vi "GUI_Frog_HPD_imagetested2.vi"() -> ()   [LabVIEW 2013]
uses:
  Shared/GUI_Template/GUI_master/tcp_new_data_event.ctl
  Shared/GUI_Template/GUI_master/tcp new data cluster.ctl
panel:
  out "tcp data event":T1
  in  "Refresh Button":bool
  in  "Select device":string(combo)="PL1-PresCtl"
  in  "triggermode::1":bool caption="Blank Button"
  out "retrievedFrogTrace::1":T2(plugin-control) caption="Retrieved Frog Trace"
  out "frogTrace::1":T2(plugin-control) caption="FROG Trace"
  in  "insert tag":bool=TRUE
  in  "stop":bool
  in  "GUIdevice 1":string="FrogHPD"
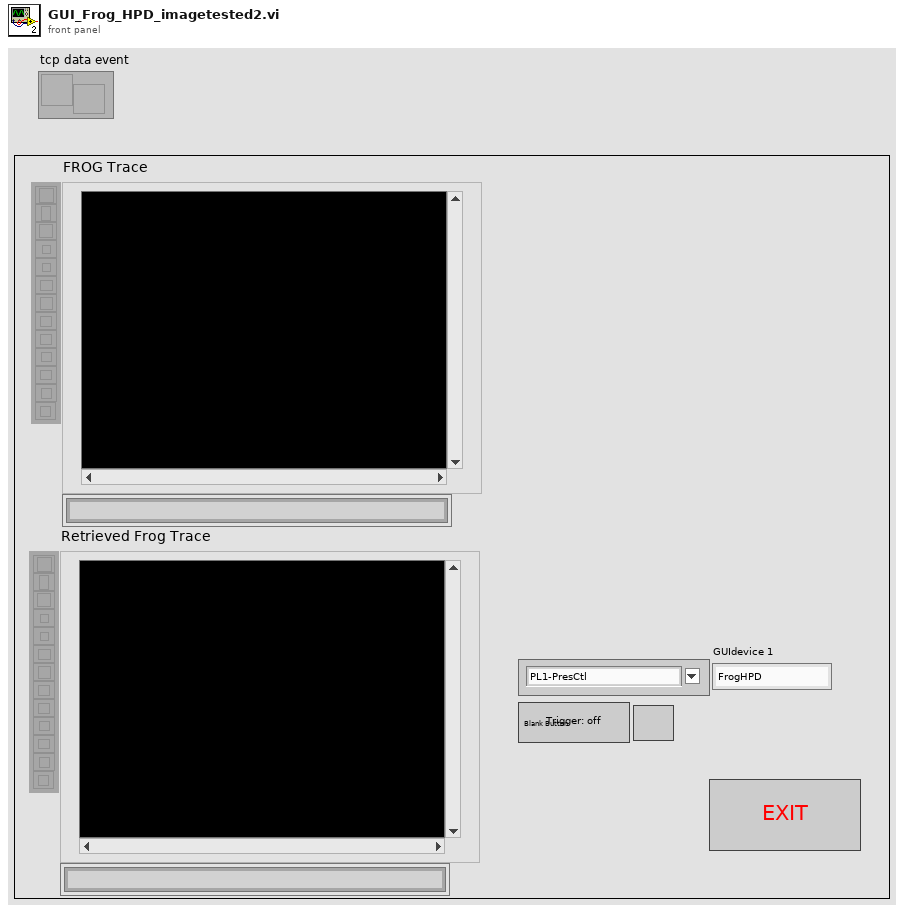
[diagram p1: front panel]
types:
  T1 = typedef "tcp_new_data_event.ctl" = refnum<user-event>
  T2 = typedef "IMAQ Image.ctl" = refnum<image>
  T3 = typedef "Image Type" = u32
  T4 = enum32{"invalid app kind", "Development System", "Run Time System", "Student Edition", "Embedded LabVIEW", "Evaluation", "Custom"}
  T5 = typedef "tcp new data cluster.ctl" = cluster{"EventEnum":enum16{"new data", "connection status update"}, "Device name":string}
  T6 = enum32{"Invalid", "Standard", "Closed", "Hidden", "Minimized", "Maximized"}
  T7 = cluster{"Core":cluster{"Current VI Reference":refnum<vi>, "Close Panel on Exit?":bool}, "Your Boolean data":bool, "Your string data":string, "SuperGUI":cluster{"STOP queue":refnum<queue>, "SuperGUI ref":refnum<vi>}}
  T8 = cluster{"STOP queue":refnum<queue>, "SuperGUI ref":refnum<vi>}
  T9 = cluster{"Current VI Reference":refnum<vi>, "Close Panel on Exit?":bool}
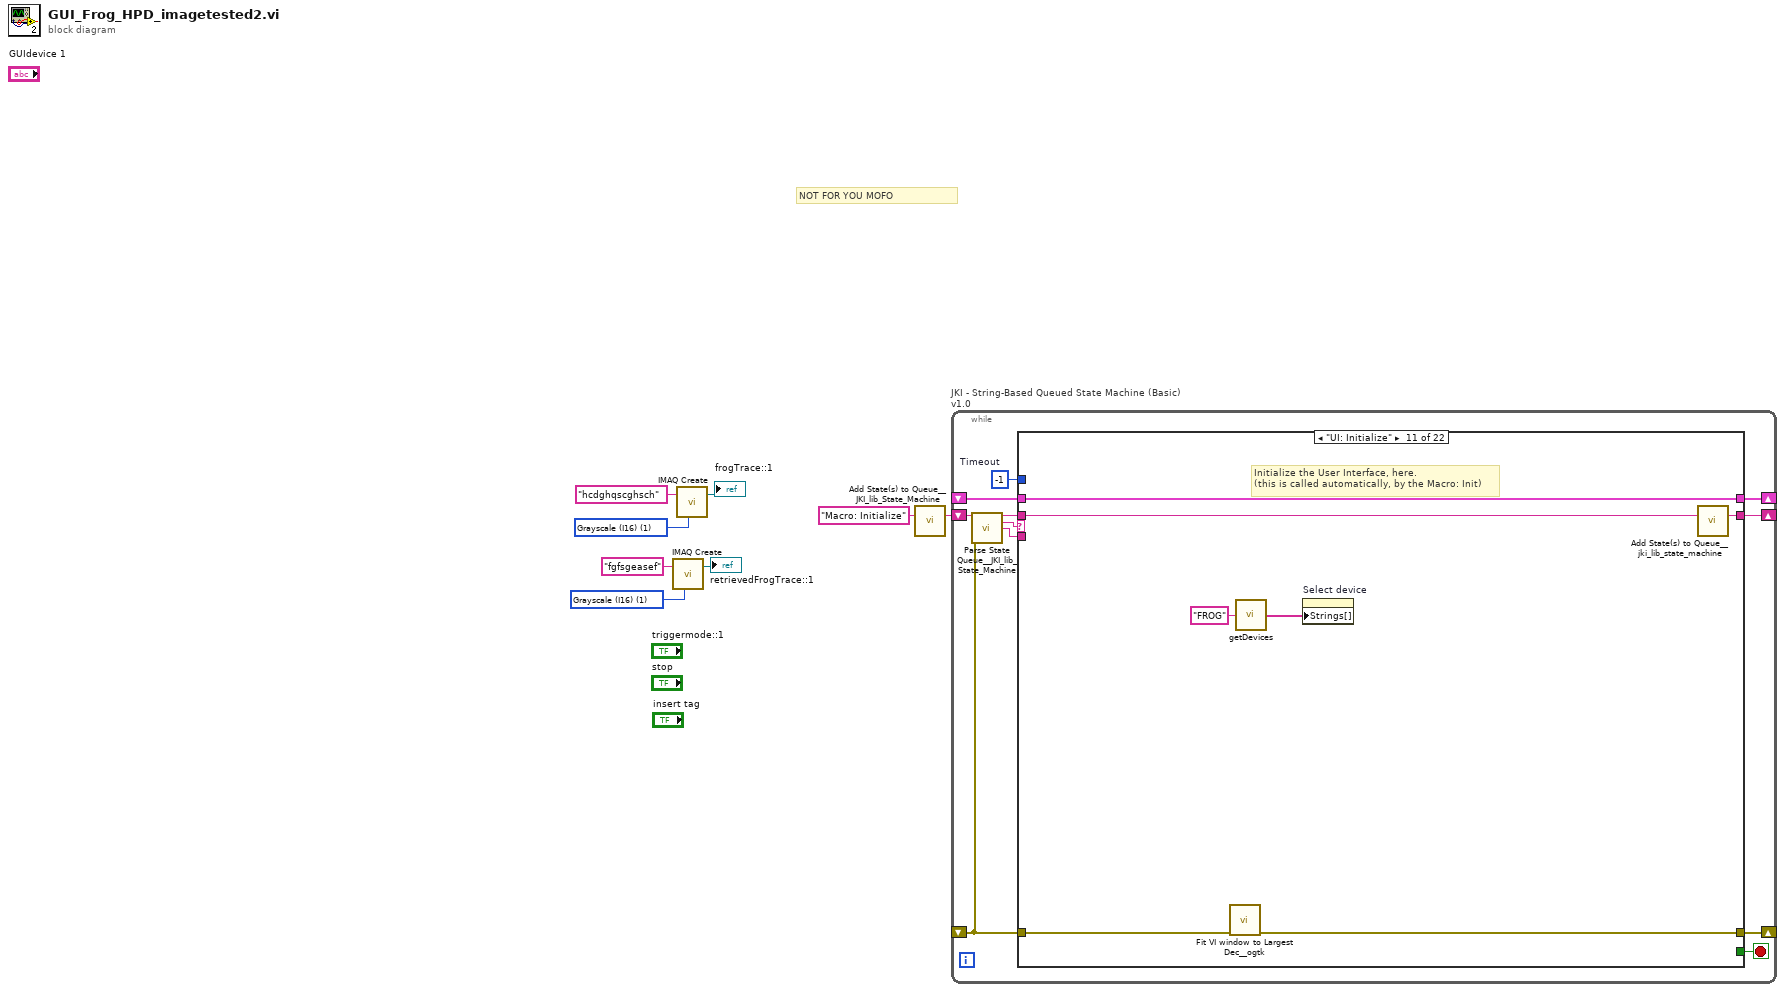
[diagram p0: block diagram]
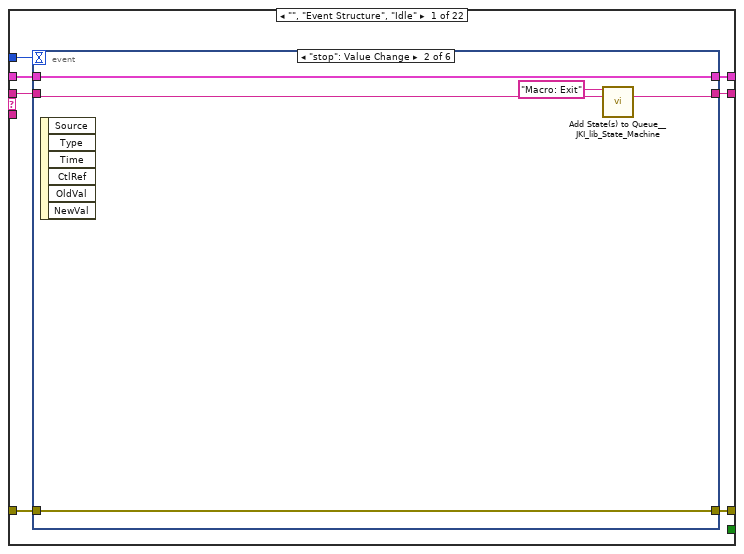
[diagram p2: hidden frame]
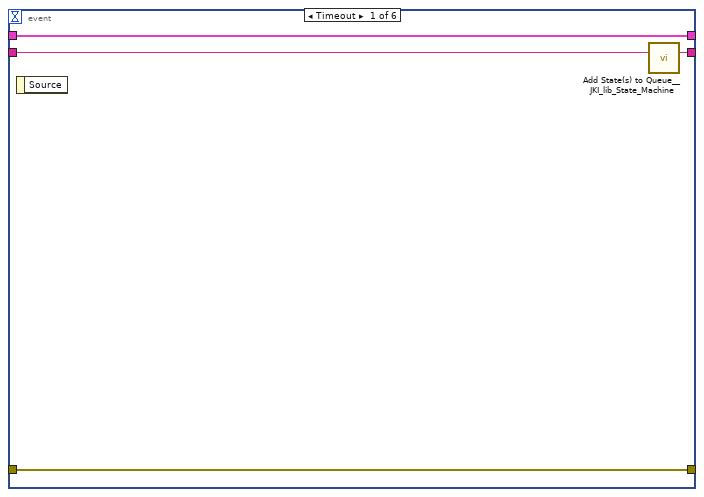
[diagram p3: hidden frame]
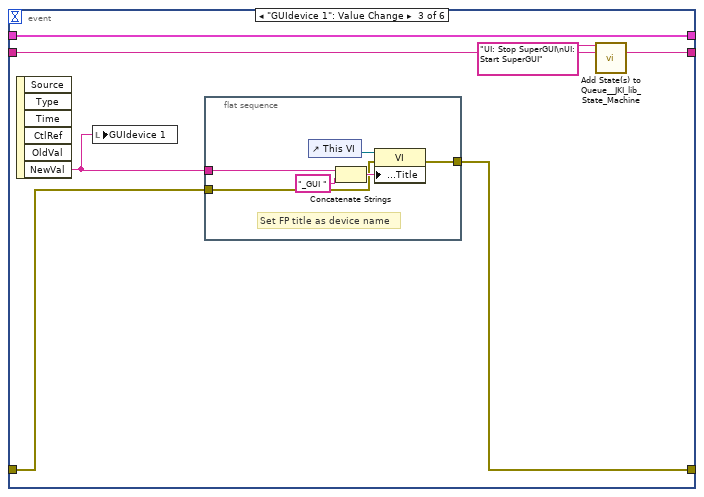
[diagram p4: hidden frame]
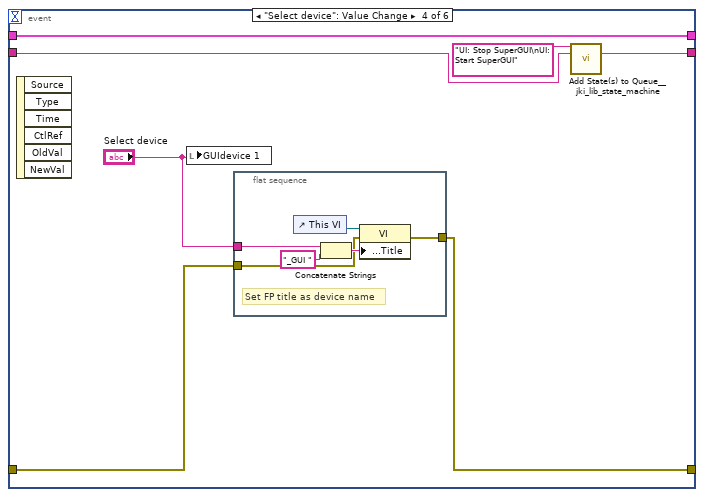
[diagram p5: hidden frame]
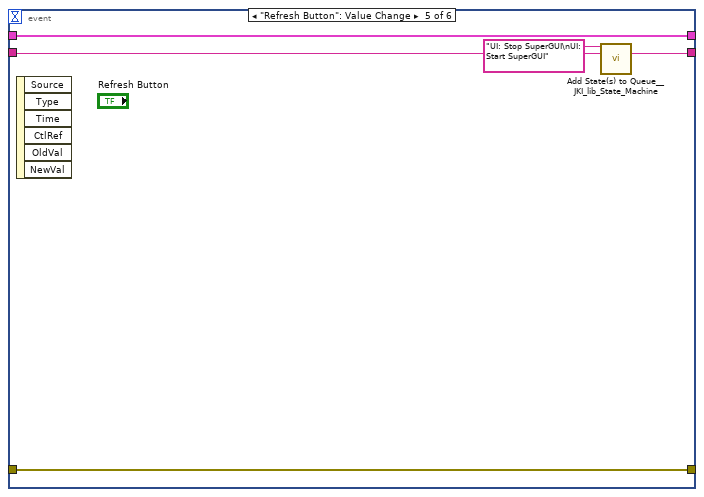
[diagram p6: hidden frame]
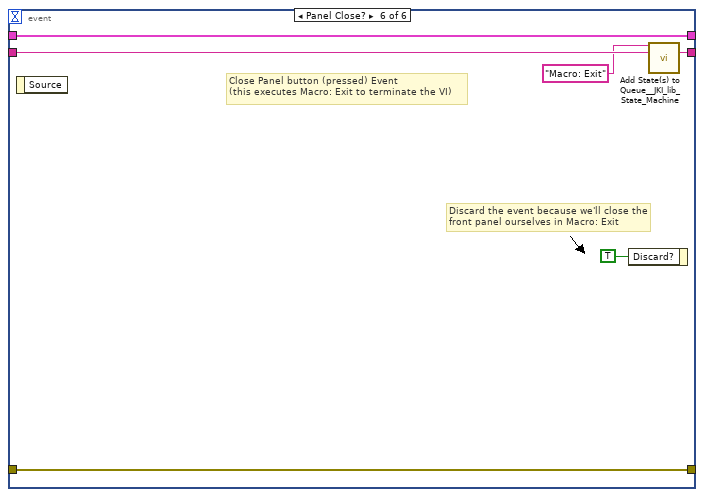
[diagram p7: hidden frame]
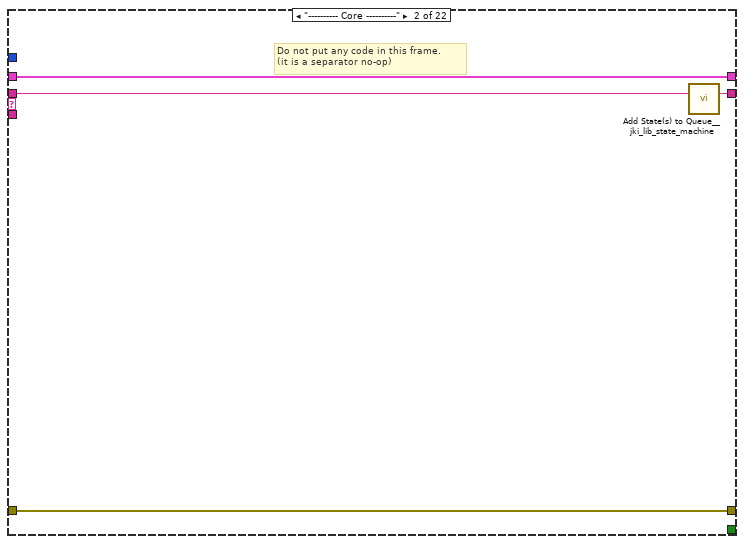
[diagram p8: hidden frame]
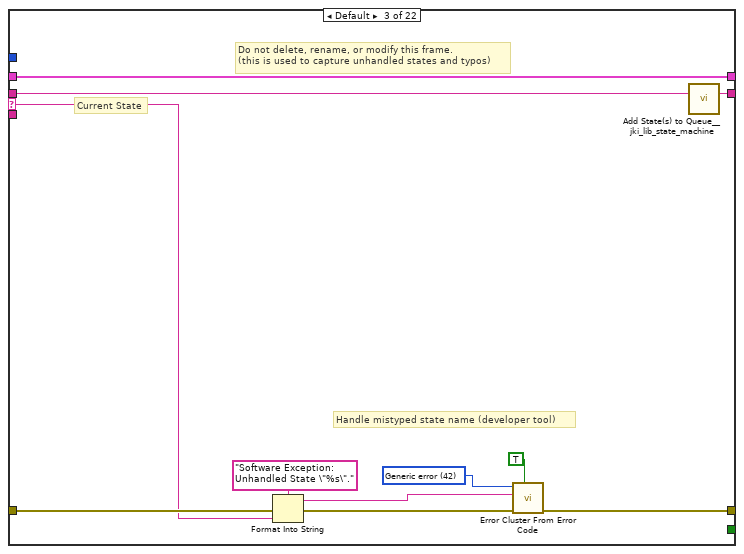
[diagram p9: hidden frame]
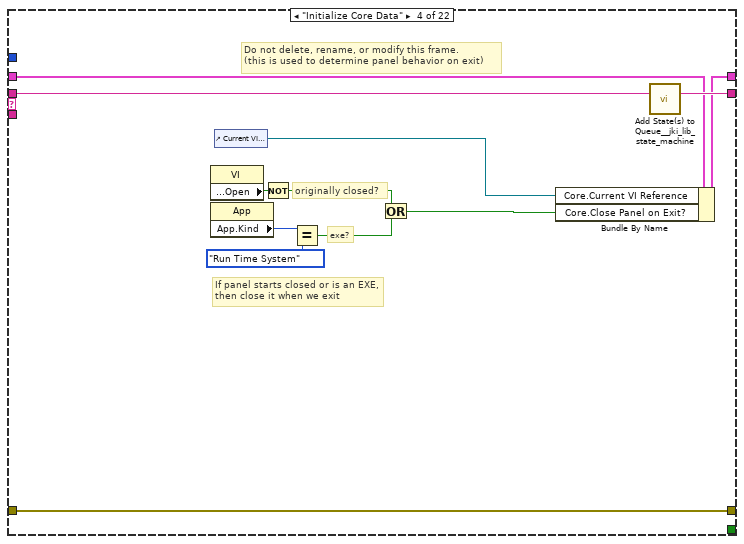
[diagram p10: hidden frame]
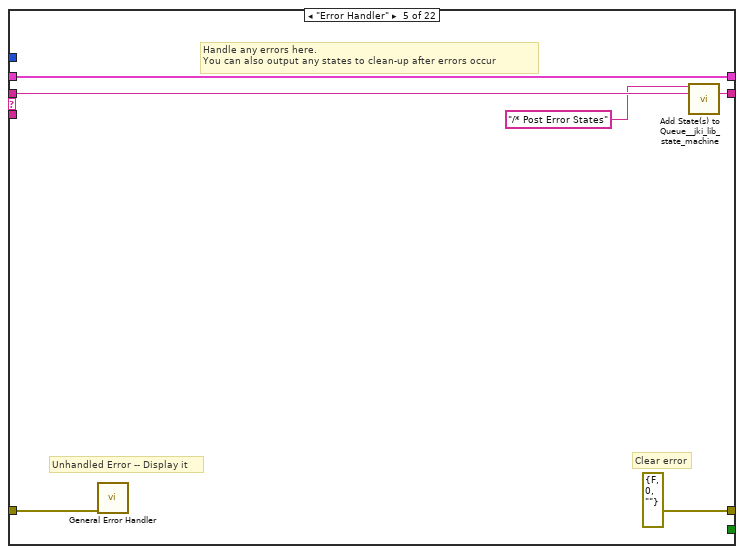
[diagram p11: hidden frame]
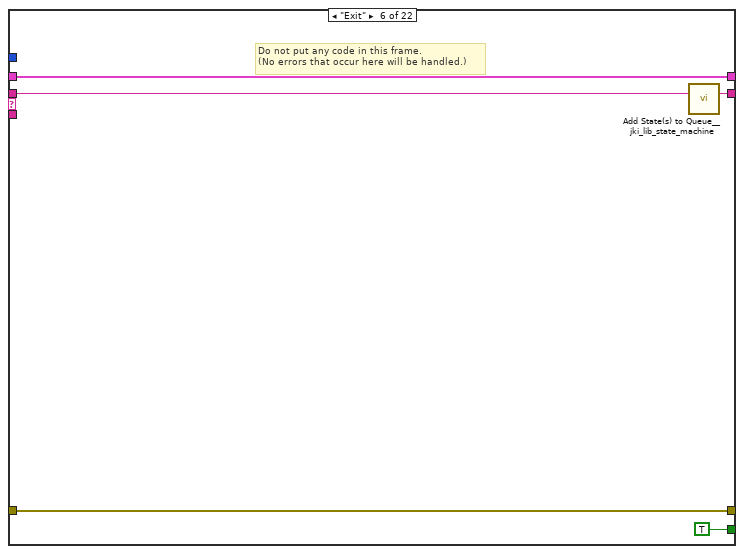
[diagram p12: hidden frame]
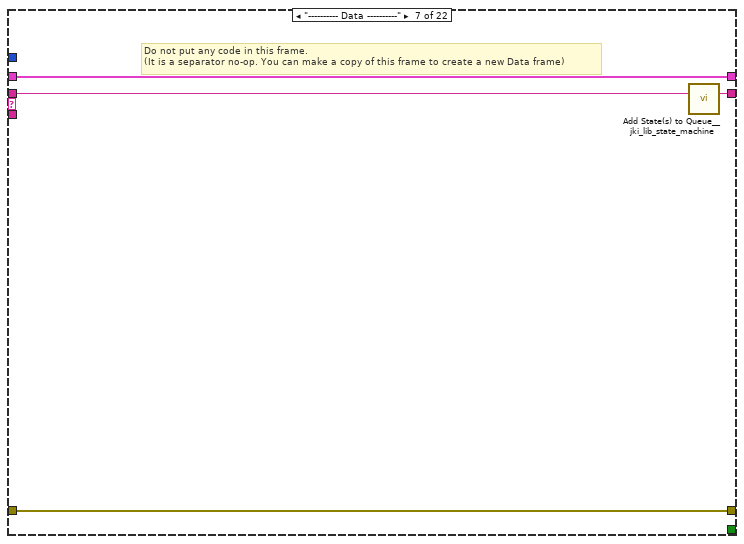
[diagram p13: hidden frame]
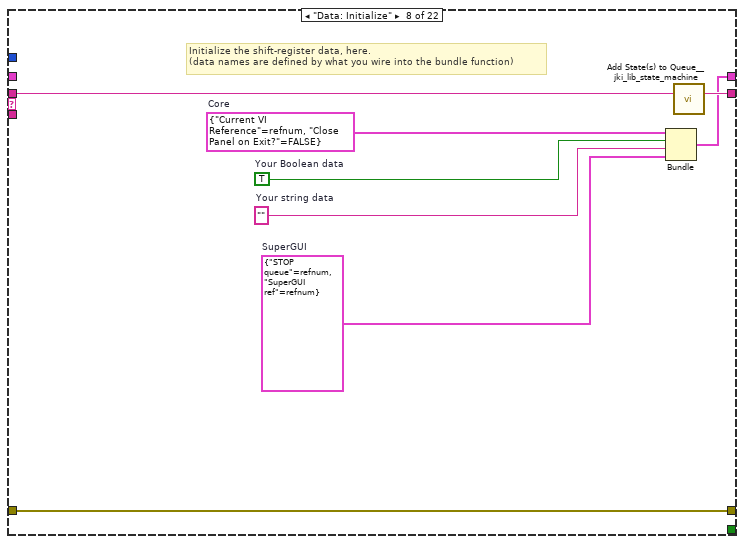
[diagram p14: hidden frame]
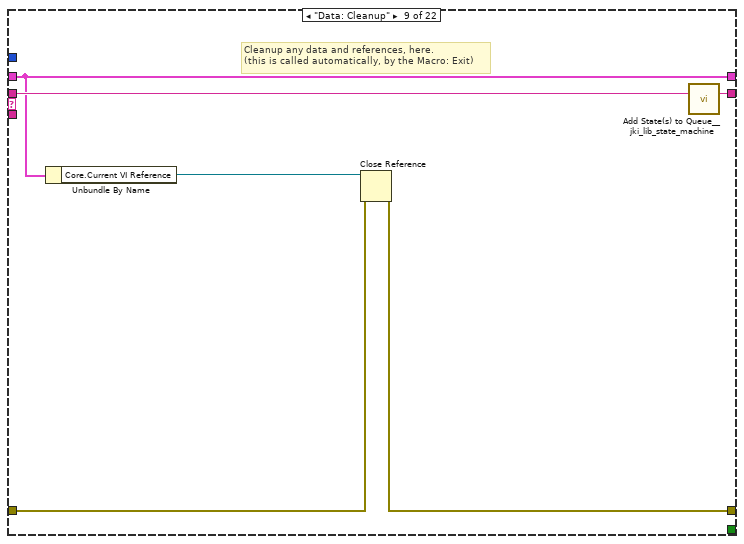
[diagram p15: hidden frame]
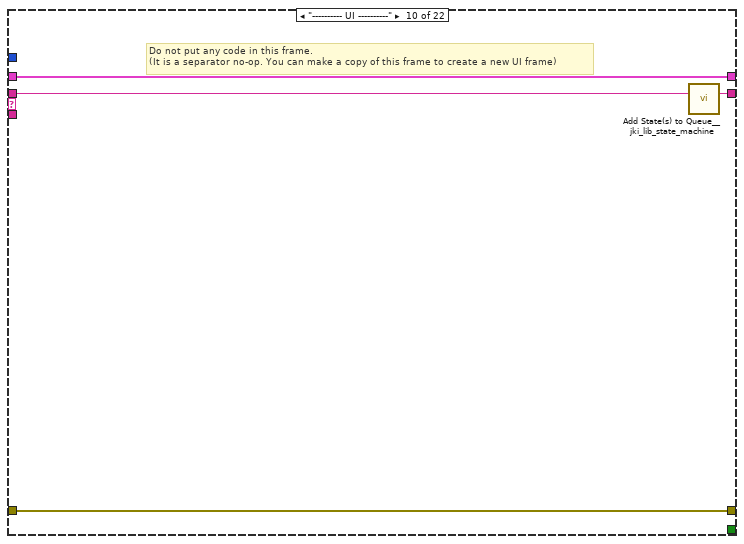
[diagram p16: hidden frame]
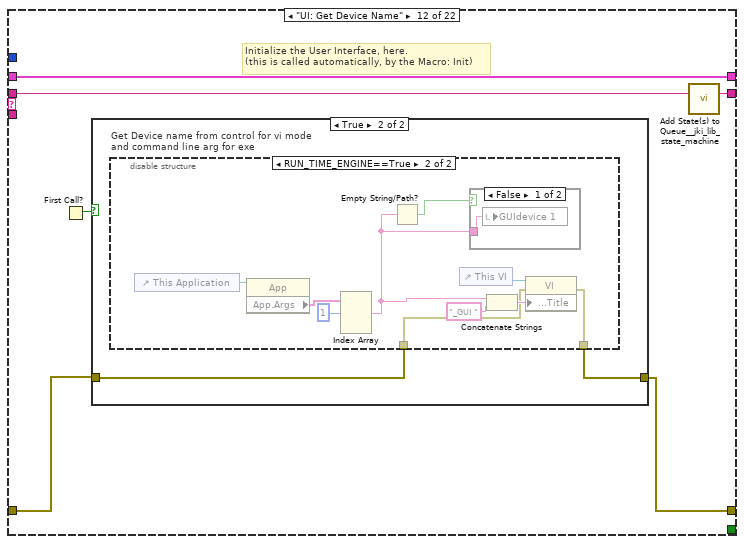
[diagram p17: hidden frame]
diagram:
  w5 = T3 1 items=["Grayscale (U8)", "Grayscale (I16)", "Grayscale (SGL)", "Complex (CSG)", "RGB (U32)", "HSL (U32)", "RGB (U64)", "Grayscale (U16)"] ("Image Type")
  w7 = T3 1 items=["Grayscale (U8)", "Grayscale (I16)", "Grayscale (SGL)", "Complex (CSG)", "RGB (U32)", "HSL (U32)", "RGB (U64)", "Grayscale (U16)"] ("Image Type")
  # "NOT FOR YOU MOFO"
  n1 = call "IMAQ Create"("Image Name"="fgfsgeasef", "Image Type"=w5) -> ("New Image"=→"retrievedFrogTrace::1":T2)  [unwired: 3 in, 1 out]
  n2 = call "IMAQ Create"("Image Name"="hcdghqscghsch", "Image Type"=w7) -> ("New Image"=→"frogTrace::1":T2)  [unwired: 3 in, 1 out]
  n3 = call <vilib>:"Add State(s) to Queue__JKI_lib_State_Machine.vi"("State(s) in (\"\")"="Macro: Initialize") -> ("States Out"=w2:string)  [unwired: 14 in]
  n4 = while "JKI - String-Based Queued State Machine (Basic) v1.0" {
    shift-right: [w12] -> _
    shift-left: _ -> [w11]
    shift-right: [w15] -> _
    shift-left: _ -> [w9]
    shift-right: [w14] -> _
    shift-left: w2 -> [w16]
    stop <- w13 stop-if-true
    w10 = -1  # Timeout
    n5 = call <vilib>:"Parse State Queue__JKI_lib_State_Machine.vi"("State Queue"=w16, "Error In (no error)"=w9) -> ("Remaining States"=w18:string, "Current State"=w19:string, "Arguments"=w17:string)  [unwired: 11 in]
    n6 = case shown="\"UI: Initialize\"" w19 {
      selector: w19 -> [_ _ w77 _ _ _ _ _ _ _ _ _ _ _ _ _ _ _ _ _ _ _]
      tunnel: w18 -> [w26 w76 w81 w99 w105 w110 w114 w122 w128 w132 w139 w145 w180 w188 w194 w205 w231 w236 w246 w250 w254 w258]
      tunnel: w17 -> [_ _ _ _ _ _ _ _ _ _ _ _ _ _ w189 w199 _ _ _ _ _ _]
      tunnel: w11 -> [w24 w73 w79 w90 w102 w108 w111 _ w123 w129 w137 w143 w171 w183 w192 w201 w228 w233 w243 w247 w251 w255]
      tunnel: [w23 w74 w83 w96 errorcluster {"status"=FALSE, "code"=0, "source"=""} ("error out") w107 w112 w119 w124 w130 w133 w140 w164 w181 w190 w202 w229 w234 w244 w248 w252 w256] -> w15
      tunnel: w9 -> [w22 w74 w82 w96 w101 w107 w112 w119 w125 w130 w136 w141 w165 w182 w191 w203 w229 w234 w244 w248 w252 w256]
      tunnel: [w25 w75 w80 w98 w104 w109 w113 w121 w127 w131 w138 w144 w179 w187 w193 w204 w230 w235 w245 w249 w253 w257] -> w14
      tunnel: [_ _ _ _ _ TRUE _ _ _ _ _ _ _ _ _ _ _ _ _ _ _ _] -> w13
      tunnel: [w21 w73 w79 w97 w102 w108 w111 w120 w123 w129 w137 w143 w170 w183 w192 w201 w228 w233 w243 w247 w251 w255] -> w12
      tunnel: w10 -> [w20 _ _ _ _ _ _ _ _ _ _ _ _ _ _ _ _ _ _ _ _ _]
      frame "", "Event Structure", "Idle" {
        n7 = event shown="[1] \"stop\": Value Change" {
          selector: _ -> [_ _ _ _ _ _]
          dyn-events: _ -> [_ _ _ _ _ _]
          timeout: w20 -> [_ _ _ _ _ _]
          tunnel: w26 -> [w30 w33 w39 w50 w64 w72]
          tunnel: [w29 w32 w38 w49 w63 w71] -> w25
          tunnel: w24 -> [w27 w35 w42 w55 w66 w69]
          tunnel: [w28 w34 w40 w52 w65 w70] -> w23
          tunnel: w22 -> [w28 w34 w41 w53 w65 w70]
          tunnel: [w27 w35 w42 w55 w66 w69] -> w21
          event Timeout {
            n8 = event-data() -> ()  [unwired: 1 in, 1 out]
            n9 = call <vilib>:"Add State(s) to Queue__JKI_lib_State_Machine.vi"("State(s) in (\"\")"=w30) -> ("States Out"=w29:string)  [unwired: 14 in]
          }
          event "stop": Value Change {
            n10 = event-data() -> ()  [unwired: 1 in, 6 out]
            n11 = call <vilib>:"Add State(s) to Queue__JKI_lib_State_Machine.vi"("State(s) in Front (\"\")"="Macro: Exit", "State(s) in (\"\")"=w33) -> ("States Out"=w32:string)  [unwired: 13 in]
          }
          event "GUIdevice 1": Value Change {
            n12 = event-data() -> ("NewVal"=w36:string)  [unwired: 1 in, 5 out]
            n13 = local write "GUIdevice 1"(w36) -> ()
            n14 = flat-sequence {
              tunnel: [w45] -> w40
              tunnel: w41 -> [w44]
              tunnel: w36 -> [w43]
              frame #0 {
                # "Set FP title as device name"
                n15 = control-ref of="This VI"() -> (w48:refnum<vi>)
                n16 = Concatenate Strings(w43, "_GUI ") -> (w47:string)
                n17 = property class="VI"(reference=w48, error in=w44, "Front Panel.Title"=w47) -> (error out=w45:errorcluster)  [unwired: 1 out]
              }
            }
            n18 = call <vilib>:"Add State(s) to Queue__JKI_lib_State_Machine.vi"("State(s) in Front (\"\")"="UI: Stop SuperGUI\nUI: Start SuperGUI", "State(s) in (\"\")"=w39) -> ("States Out"=w38:string)  [unwired: 13 in]
          }
          event "Select device": Value Change {
            n19 = event-data() -> ()  [unwired: 1 in, 6 out]
            n20 = local write "GUIdevice 1"("Select device") -> ()
            n21 = flat-sequence {
              tunnel: [w58] -> w52
              tunnel: w53 -> [w57]
              tunnel: "Select device" -> [w56]
              frame #0 {
                # "Set FP title as device name"
                n22 = control-ref of="This VI"() -> (w61:refnum<vi>)
                n23 = Concatenate Strings(w56, "_GUI ") -> (w60:string)
                n24 = property class="VI"(reference=w61, error in=w57, "Front Panel.Title"=w60) -> (error out=w58:errorcluster)  [unwired: 1 out]
              }
            }
            n25 = call <vilib>:"Add State(s) to Queue__jki_lib_state_machine.vi"("State(s) in Front (\"\")"="UI: Stop SuperGUI\nUI: Start SuperGUI", "State(s) in (\"\")"=w50) -> ("States Out"=w49:string)  [unwired: 13 in]
          }
          event "Refresh Button": Value Change {
            n26 = event-data() -> ()  [unwired: 1 in, 6 out]
            n27 = call <vilib>:"Add State(s) to Queue__JKI_lib_State_Machine.vi"("State(s) in Front (\"\")"="UI: Stop SuperGUI\nUI: Start SuperGUI", "State(s) in (\"\")"=w64) -> ("States Out"=w63:string)  [unwired: 13 in]
          }
          event Panel Close? {
            # "Discard the event because we'll close the front panel ourselves in Macro: Exit"
            # "Close Panel button (pressed) Event\n(this executes Macro: Exit to terminate the VI)"
            n28 = event-data() -> ()  [unwired: 1 in, 1 out]
            n29 = event-data("Discard?"=TRUE) -> ()  [unwired: 1 in, 1 out]
            n30 = call <vilib>:"Add State(s) to Queue__JKI_lib_State_Machine.vi"("State(s) in Front (\"\")"="Macro: Exit", "State(s) in (\"\")"=w72) -> ("States Out"=w71:string)  [unwired: 13 in]
          }
        }
      }
      frame "---------- Core ----------" {
        # "Do not put any code in this frame.\n(it is a separator no-op)"
        n31 = call <vilib>:"Add State(s) to Queue__jki_lib_state_machine.vi"("State(s) in (\"\")"=w76) -> ("States Out"=w75:string)  [unwired: 14 in]
      }
      frame Default {
        w86 = 42 items=["No error", "Argument error", "Memory is full", "Out of zone", "End of file", "File already open", "Generic file I/O error", "File not found", "File permission error", "Disk is full", "Duplicate path", "Too many files open", "System feature not enabled", "Resource file not found", "Cannot add resource", "Resource not found", "Image not found", "Image memory error", "Pen does not exist", "Config type invalid", "Config token not found", "Config parse error", "Config memory error", "Bad external code format", "Bad external code offset", "External code not present", "Null window", "Destroy window error", "Null menu", "Print aborted", "Bad print record", "Print driver error", "Windows error during printing", "Memory error during printing", "Print dialog error", "Generic print error", "Invalid device refnum", "Device not found", "Device parameter error", "Device unit error", "Cannot open device", "Device call aborted", "Generic error", "Cancelled by user", "Object ID too low", "Object ID too high", "Object not in heap", "Unknown heap", "Unknown object (invalid DefProc)", "Unknown object (DefProc not in table)", "Message out of range", "Invalid (null) method", "Unknown message", "Manager call not supported", "Bad address", "Network operation in progress", "Network operation timed out", "Connection is busy", "Network attribute not supported", "Network error", "Address in use", "System out of memory", "Connection aborted", "Connection refused", "Not connected", "Already connected", "Connection closed", "Initialization error (interapplication manager)", "Bad occurrence", "Wait on unbound occurrence handler", "Occurrence queue overflow", "Datalog type conflict", "Unused", "Unrecognized type (interapplication manager)", "Memory corrupt", "Failed to make temporary DLL", "Old CIN version", "Drag socket not found", "Failed to load drop-object", "Failed to register OLE object", "Failed to release OLE object", "Format specifier type mismatch", "Unknown format specifier", "Too few format specifiers", "Too many format specifiers", "Scan failed", "Newer CIN version", "Error converting to variant", "Runtime menu error", "Password tampered", "Variant attribute not found", "Incompatible variant data type", "Event data is not available", "Event Store is not present", "Occurrence is not found", "Event Queue is not created", "Event info is not available", "Refnum passed is NULL", "Error retrieving Class GUID", "Error retrieving CoClass GUID", "Error retrieving TypeLib GUID.", "Bad built application magic bytes.", "Specific driver is different from the specific driver associated with the Logical Name.", "There is no session opened to the class driver.", "Max Error", "MAX - Error with config objects", "MAX - Error loading configuration", "MAX - Group not supported"]
        # "Current State"
        # "Do not delete, rename, or modify this frame.\n(this is used to capture unhandled states and typos)"
        # "Handle mistyped state name (developer tool)"
        n32 = Format Into String(format string="Software Exception: Unhandled State \"%s\"." ("message"), error in=w82, w77) -> (resulting string=w85:string, error out=w84:errorcluster)  [unwired: 1 in]
        n33 = call <vilib>:"Error Cluster From Error Code.vi"("show call chain? (False)"=TRUE, "error in (no error)"=w84, "error message (\"\")"=w85, "error code (0)"=w86) -> ("error out"=w83:errorcluster)  [unwired: 5 in]
        n34 = call <vilib>:"Add State(s) to Queue__jki_lib_state_machine.vi"("State(s) in (\"\")"=w81) -> ("States Out"=w80:string)  [unwired: 14 in]
      }
      frame "Initialize Core Data" {
        # "Do not delete, rename, or modify this frame.\n(this is used to determine panel behavior on exit)"
        # "originally closed?"
        # "exe?"
        # "If panel starts closed or is an EXE, then close it when we exit"
        n35 = property class="VI"() -> ("Front Panel.Open"=w95:bool)  [unwired: 2 in, 2 out]
        n36 = property class="App"() -> ("App.Kind"=w94:T4)  [unwired: 2 in, 2 out]
        n37 = control-ref of="Current VI Reference"() -> (w88:refnum<vi>)
        n38 = Not(x=w95) -> (.not. x?=w92:bool)
        n39 = Equal?(x=w94, y=T4."Run Time System" ("Application:Kind")) -> (x = y?=w91:bool)
        n40 = Or(x=w92, y=w91) -> (x .or. y?=w89:bool)
        n41 = Bundle By Name(cluster=w90, "Core.Current VI Reference"=w88, "Core.Close Panel on Exit?"=w89) -> (w97:T7)
        n42 = call <vilib>:"Add State(s) to Queue__jki_lib_state_machine.vi"("State(s) in (\"\")"=w99) -> ("States Out"=w98:string)  [unwired: 14 in]
      }
      frame "Error Handler" {
        # "Unhandled Error -- Display it"
        # "Handle any errors here.\nYou can also output any states to clean-up after errors occur"
        # "Clear error"
        n43 = call <vilib>:"General Error Handler.vi"("error in (no error)"=w101) -> ()  [unwired: 10 in, 5 out]
        n44 = call <vilib>:"Add State(s) to Queue__jki_lib_state_machine.vi"("State(s) in Front (\"\")"="/* Post Error States", "State(s) in (\"\")"=w105) -> ("States Out"=w104:string)  [unwired: 13 in]
      }
      frame "Exit" {
        # "Do not put any code in this frame.\n(No errors that occur here will be handled.)"
        n45 = call <vilib>:"Add State(s) to Queue__jki_lib_state_machine.vi"("State(s) in (\"\")"=w110) -> ("States Out"=w109:string)  [unwired: 14 in]
      }
      frame "---------- Data ----------" {
        # "Do not put any code in this frame.\n(It is a separator no-op. You can make a copy of this frame to create a new Data frame)"
        n46 = call <vilib>:"Add State(s) to Queue__jki_lib_state_machine.vi"("State(s) in (\"\")"=w114) -> ("States Out"=w113:string)  [unwired: 14 in]
      }
      frame "Data: Initialize" {
        w115 = T8 {"STOP queue"=refnum, "SuperGUI ref"=refnum}  # SuperGUI
        w116 = T9 {"Current VI Reference"=refnum, "Close Panel on Exit?"=FALSE}  # Core
        w118 = TRUE  # Your Boolean data
        w117 = ""  # Your string data
        # "Initialize the shift-register data, here.\n(data names are defined by what you wire into the bundle function)"
        n47 = Bundle("Core"=w116, "Your Boolean data"=w118, "Your string data"=w117, "SuperGUI"=w115) -> (w120:T7)  [unwired: 1 in]
        n48 = call <vilib>:"Add State(s) to Queue__jki_lib_state_machine.vi"("State(s) in (\"\")"=w122) -> ("States Out"=w121:string)  [unwired: 14 in]
      }
      frame "Data: Cleanup" {
        # "Cleanup any data and references, here.\n(this is called automatically, by the Macro: Exit)"
        n49 = Unbundle By Name(w123) -> ("Core.Current VI Reference"=w126:refnum<vi>)
        n50 = Close Reference(reference=w126, error in (no error)=w125) -> (error out=w124:errorcluster)
        n51 = call <vilib>:"Add State(s) to Queue__jki_lib_state_machine.vi"("State(s) in (\"\")"=w128) -> ("States Out"=w127:string)  [unwired: 14 in]
      }
      frame "---------- UI ----------" {
        # "Do not put any code in this frame.\n(It is a separator no-op. You can make a copy of this frame to create a new UI frame)"
        n52 = call <vilib>:"Add State(s) to Queue__jki_lib_state_machine.vi"("State(s) in (\"\")"=w132) -> ("States Out"=w131:string)  [unwired: 14 in]
      }
      frame "UI: Initialize" {
        # "Initialize the User Interface, here.\n(this is called automatically, by the Macro: Init)"
        n53 = call <userlib>:"Fit VI window to Largest Dec__ogtk.vi"("error in (no error)"=w136) -> ("error out"=w133:errorcluster)  [unwired: 5 in, 1 out]
        n54 = call "getDevices.vi"("Device Class"="FROG") -> ("All Devices"=w134:string[])
        n55 = property on="Select device" class="CmbBox"("Strings[]"=w134) -> ()  [unwired: 2 in, 2 out]
        n56 = call <vilib>:"Add State(s) to Queue__jki_lib_state_machine.vi"("State(s) in (\"\")"=w139) -> ("States Out"=w138:string)  [unwired: 14 in]
      }
      frame "UI: Get Device Name" {
        # "Initialize the User Interface, here.\n(this is called automatically, by the Macro: Init)"
        n57 = First Call?() -> (First Call?: T/F=w142:bool)
        n58 = case shown="True" w142 {
          tunnel: w141 -> [w146 w148]
          tunnel: [w146 w147] -> w140
          frame False {
          }
          frame True {
            n59 = disable-structure "Get Device name from control for vi mode\nand command line arg for exe" shown="RUN_TIME_ENGINE==True" {
              disable-tunnel: w148 -> [w149 w151]
              disable-tunnel: [w149 w150] -> w147
              frame condition #0 (active) {
              }
              frame condition #1 {
                n60 = control-ref of="This Application"() -> (w159:refnum<vi>)
                n61 = property class="App"(reference=w159) -> ("App.Args"=w158:string[])  [unwired: 1 in, 2 out]
                n62 = Index Array(array=w158, index #1=1 ("index")) -> (element #1=w152:string)  [unwired: 2 in, 2 out]
                n63 = Empty String/Path?(string/path=w152) -> (empty?=w156:bool)
                n64 = control-ref of="This VI"() -> (w155:refnum<vi>)
                n65 = case shown="False" w156 {
                  tunnel: w152 -> [w160 _]
                  frame False {
                    n66 = local write "GUIdevice 1"(w160) -> ()
                  }
                  frame True {
                  }
                }
                n67 = Concatenate Strings(w152, "_GUI ") -> (w154:string)
                n68 = property class="VI"(reference=w155, error in=w151, "Front Panel.Title"=w154) -> (error out=w150:errorcluster)  [unwired: 1 out]
              }
            }
          }
        }
        n69 = call <vilib>:"Add State(s) to Queue__jki_lib_state_machine.vi"("State(s) in (\"\")"=w145) -> ("States Out"=w144:string)  [unwired: 14 in]
      }
      frame "UI: Start SuperGUI" {
        # "create stop queue for supergui and its clones"
        # "x100 abort will be dependent on caller VI\nx80 abort will be independent of caller vi, this will abort vi when labview is closed."
        # "Start SuperGUI asynchronous way"
        n70 = vi-ref "GUI_Master_subvi_reentrant_queues.vi"() -> (w163:refnum<vi>)
        n71 = property class="VI"(reference=w163) -> ("Path"=w162:path)  [unwired: 1 in, 2 out]
        n72 = Create User Event(user event datatype=T5 {"EventEnum"=enum."new data", "Device name"="Device name"} ("New Event"), error in=w165) -> (user event=w166:refnum<user-event>, error out=w172:errorcluster)
        "tcp data event" <- w166
        n73 = control-ref of="This Application"() -> (w169:refnum<vi>)
        n74 = control-ref of="This VI"() -> (w168:refnum<vi>)
        n75 = Open VI Reference(type specifier VI Refnum (for type only)=refnum<vi> refnum, vi path=w162, options=256) -> (vi reference=w178:refnum<vi>, error out=w177:errorcluster)  [unwired: 3 in]
        n76 = register-events(w166) -> ()  [unwired: 2 in, 2 out]
        n77 = call "supergui create stop queue.vi"() -> ("STOP Queue out"=w174:refnum<queue>)  [unwired: 11 in]
        n78 = Current VI's Menubar() -> (w167:refnum<k9>)
        n79 = call-by-ref "Start Asynchronous Call"(reference=w178, error in=w177, "STOP Queue in"=w174, "This Application"=w169, 8:"error in (no error)"=w172, "tcp data event"=w166, "Caller menu reference"=w167, "Caller VI ref"=w168) -> (reference out=w161:refnum<vi>, error out=w164:errorcluster)  [unwired: 5 in, 1 out]
        n80 = Bundle By Name(cluster=w171, "SuperGUI.SuperGUI ref"=w161, "SuperGUI.STOP queue"=w174) -> (w170:T7)
        n81 = call <vilib>:"Add State(s) to Queue__jki_lib_state_machine.vi"("State(s) in (\"\")"=w180) -> ("States Out"=w179:string)  [unwired: 14 in]
      }
      frame "UI: Stop SuperGUI" {
        # "Stop Supergui Clone and wait until it exit properly"
        n82 = Unbundle By Name(w183) -> ("SuperGUI.SuperGUI ref"=w185:refnum<vi>, "SuperGUI.STOP queue"=w184:refnum<queue>)
        n83 = Release Queue(queue=w184, error in (no error)=w182) -> (error out=w186:errorcluster)  [unwired: 1 in, 2 out]
        n84 = call-by-ref "Wait On Asynchronous Call"(reference=w185, error in=w186) -> ("error out"=w181:errorcluster)  [unwired: 11 in, 2 out]
        n85 = call <vilib>:"Add State(s) to Queue__jki_lib_state_machine.vi"("State(s) in (\"\")"=w188) -> ("States Out"=w187:string)  [unwired: 14 in]
      }
      frame "UI: Cursor Set" {
        # "Argument"
        # "Set and Unset Cursor Busy.\n(Usage: \"UI: Cursor Set >> Busy|Idle\")"
        n86 = case shown="\"Idle\", Default" w189 {
          tunnel: w191 -> [w196 w198]
          tunnel: [w195 w197] -> w190
          frame "Idle", Default {
            n87 = call <vilib>:"Unset Busy.vi"("error in (no error)"=w196) -> ("error out"=w195:errorcluster)  [unwired: 10 in]
          }
          frame "Busy" {
            n88 = call <vilib>:"Set Busy.vi"("error in (no error)"=w198) -> ("error out"=w197:errorcluster)  [unwired: 9 in, 1 out]
          }
        }
        n89 = call <vilib>:"Add State(s) to Queue__jki_lib_state_machine.vi"("State(s) in (\"\")"=w194) -> ("States Out"=w193:string)  [unwired: 14 in]
      }
      frame "UI: Front Panel State" {
        # "Argument"
        # "Set Front Panel Open or Closed\n(Usage: \"UI: Front Panel State >> Open|Close\")"
        n90 = Unbundle By Name(w201) -> ("Core.Current VI Reference"=w200:refnum<vi>)
        n91 = case shown="\"Open\", Default" w199 {
          tunnel: w203 -> [w209 w222]
          tunnel: [w211 w223] -> w202
          tunnel: w200 -> [w210 w220]
          frame "Open", Default {
            n92 = property class="VI"(reference=w210, error in=w209) -> (reference out=w207:refnum<vi>, error out=w208:errorcluster, "Front Panel.Open"=w206:bool)
            n93 = case shown="False" w206 {
              tunnel: [w214 w217] -> w211
              tunnel: w208 -> [w213 w217]
              tunnel: w207 -> [w212 _]
              frame False {
                n94 = invoke class="VI" method="FP.Open"(reference=w212, error in=w213, "Activate"=TRUE, "State"=T6."Standard") -> (error out=w214:errorcluster)  [unwired: 1 in, 4 out]
              }
              frame True {
              }
            }
          }
          frame "Close" {
            n95 = property class="VI"(reference=w220, error in=w222) -> (reference out=w219:refnum<vi>, error out=w221:errorcluster, "Front Panel.Open"=w218:bool)
            n96 = case shown="True" w218 {
              tunnel: [w224 w227] -> w223
              tunnel: w221 -> [w224 w226]
              tunnel: w219 -> [_ w225]
              frame False {
              }
              frame True {
                n97 = invoke class="VI" method="FP.Close"(reference=w225, error in=w226) -> (error out=w227:errorcluster)  [unwired: 1 in, 2 out]
              }
            }
          }
        }
        n98 = call <vilib>:"Add State(s) to Queue__jki_lib_state_machine.vi"("State(s) in (\"\")"=w205) -> ("States Out"=w204:string)  [unwired: 14 in]
      }
      frame "---------- Macro ----------" {
        # "Do not put any code in this frame.\n(It is a separator no-op. You can make a copy of this frame to create a new Macro frame)"
        n99 = call <vilib>:"Add State(s) to Queue__jki_lib_state_machine.vi"("State(s) in (\"\")"=w231) -> ("States Out"=w230:string)  [unwired: 14 in]
      }
      frame "Macro: Initialize" {
        # "Initialization Macro\n(This is called once, when the VI starts)"
        n100 = call <vilib>:"Add State(s) to Queue__jki_lib_state_machine.vi"("State(s) in Front (\"\")"="Data: Initialize\nInitialize Core Data\nUI: Initialize\nUI: Get Device Name\nUI: Start SuperGUI\nUI: Front Panel State >> Open", "State(s) in (\"\")"=w236) -> ("States Out"=w235:string)  [unwired: 13 in]
      }
      frame "Macro: Exit" {
        # "Exit Macro\n(This is called once, when the VI exits)"
        n101 = Unbundle By Name(w243) -> ("Core.Close Panel on Exit?"=w242:bool)
        n102 = Select(t="UI: Front Panel State >> Close", s=w242, f="") -> (s? t:f=w239:string)
        n103 = call <vilib>:"Add State(s) to Queue__jki_lib_state_machine.vi"("State(s) in (\"\")"=w239, "State(s) at Back (\"\")"="Data: Cleanup\nExit") -> ("States Out"=w237:string)  [unwired: 13 in]
        n104 = call <vilib>:"Add State(s) to Queue__jki_lib_state_machine.vi"("State(s) in Front (\"\")"=w237, "State(s) in (\"\")"=w246) -> ("States Out"=w245:string)  [unwired: 13 in]
      }
      frame "---------- New Category ----------" {
        # "Template Separator\n(You can make a copy of, or modify, this frame)"
        n105 = call <vilib>:"Add State(s) to Queue__jki_lib_state_machine.vi"("State(s) in (\"\")"=w250) -> ("States Out"=w249:string)  [unwired: 14 in]
      }
      frame "New Category: 1" {
        # "Your code here.\n(You can make a copy of, or modify, this frame)"
        n106 = call <vilib>:"Add State(s) to Queue__jki_lib_state_machine.vi"("State(s) in (\"\")"=w254) -> ("States Out"=w253:string)  [unwired: 14 in]
      }
      frame "New Category: 2" {
        # "Your code here.\n(You can make a copy of, or modify, this frame)"
        n107 = call <vilib>:"Add State(s) to Queue__jki_lib_state_machine.vi"("State(s) in (\"\")"=w258) -> ("States Out"=w257:string)  [unwired: 14 in]
      }
    }
  }
